vi "Initialize_system.vi"(10 "Serial Port":refnum<visa-resource-name>="COM8", 11 "String in":refnum<vi>) -> (0 "error out":errorcluster, 2 "error?":bool, 3 "VISA Refnum out":refnum<visa-resource-name>, 4 "Results_dir":path)   [LabVIEW 2019]
uses:
  <vilib>/Utility/error.llb/DialogType.ctl
  <vilib>/Instr/_visa.llb/VISA Configure Serial Port (Instr).vi
  Board_Global_Var.vi
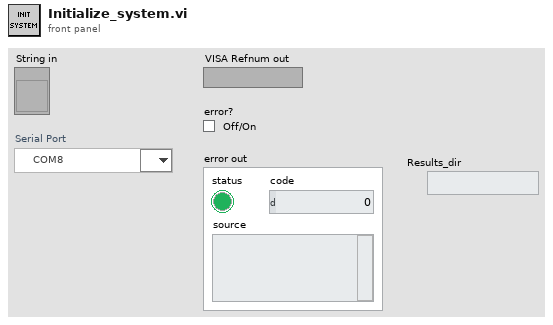
[diagram p1: front panel]
types:
  T1 = typedef "DialogType.ctl" = u16
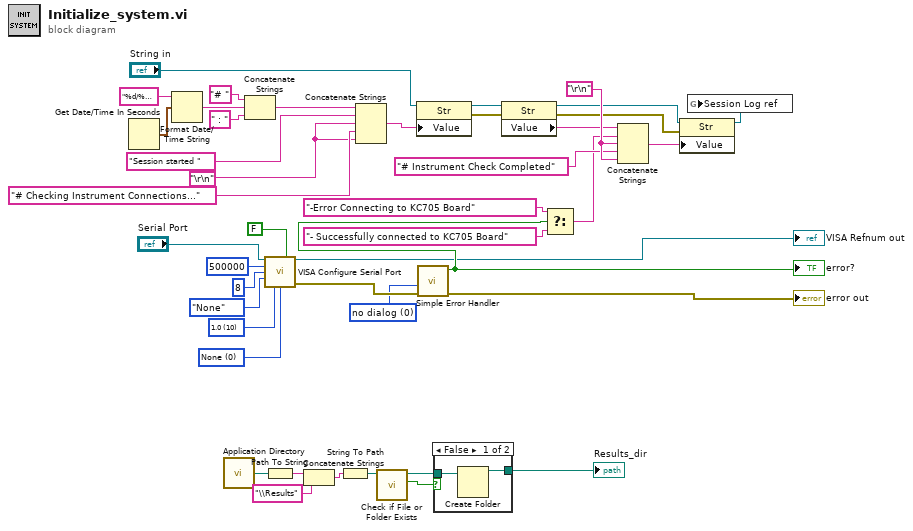
[diagram p0: block diagram]
diagram:
  w34 = u16 0 items=["None", "XON/XOFF", "RTS/CTS", "XON/XOFF & RTS/CTS", "DTR/DSR", "XON/XOFF & DTR/DSR"] ("flow control (0:none)")
  w33 = u16 10 items=["1.0"=10, "1.5"=15, "2.0"=20] ("stop bits (10: 1 bit)")
  w37 = "\r\n"
  w23 = T1 0 items=["no dialog", "OK message", "continue or stop message", "OK message + warnings", "continue/stop + warnings"] ("type of dialog (OK msg:1)")
  w13 = "\r\n"
  n1 = Get Date/Time In Seconds() -> (seconds since 1Jan1904=w19:timestamp)
  n2 = Format Date/Time String(time format string (%c)="%d/%m/%y_%H:%M:%S", seconds (now)=w19) -> (date/time string=w17:string)  [unwired: 1 in]
  n3 = call <vilib>:"Application Directory.vi"() -> ("Application Directory"=w3:path)
  n4 = Concatenate Strings("# " ("string"), w17, " : " ("string")) -> (w16:string)
  n5 = call-poly "VISA Configure Serial Port"("VISA resource name"="Serial Port", "Enable Termination\nChar (T)"=FALSE ("Enable Termination\nChar (T)"), "baud rate (9600)"=u32 500000, "data bits (8)"=u16 8, "parity (0:none)"=enum16{"None", "Odd", "Even", "Mark", "Space"}."None", "stop bits (10: 1 bit)"=w33, "flow control (0:none)"=w34) -> ("VISA resource name out"=→"VISA Refnum out":refnum<visa-resource-name>, "error out"=w38:errorcluster)  [unwired: 7 in]
  n6 = Path To String(path=w3) -> (string=w2:string)
  n7 = Concatenate Strings(w2, "\\Results" ("string")) -> (w8:string)
  n8 = String To Path(string=w8) -> (path=w7:path)
  n9 = Concatenate Strings(w16, "Session started ", w13, "# Checking Instrument Connections..." ("string"), w13) -> (w12:string)
  n10 = call <vilib>:"Check if File or Folder Exists.vi"("path"=w7) -> ("file or folder exists?"=w6:bool, "dup path"=w5:path)  [unwired: 8 in, 1 out]
  n11 = property on="Property Node" class="Str"(reference="String in", "Value"=w12) -> (reference out=w11:refnum<vi>, error out=w10:errorcluster)  [unwired: 1 in]
  n12 = call <vilib>:"Simple Error Handler.vi"("type of dialog (OK msg:1)"=w23, "error in (no error)"=w38) -> ("error?"=w43:bool, "error out"=→"error out":errorcluster)  [unwired: 3 in, 3 out]
  "error?" <- w43
  n13 = case shown="False" w6 {
    tunnel: [w45 w46] -> w1
    tunnel: w5 -> [w44 w46]
    frame False {
      n14 = Create Folder(path (use dialog)=w44) -> (created path=w45:path)  [unwired: 2 in, 2 out]
    }
    frame True {
    }
  }
  "Results_dir" <- w1
  n15 = property on="Property Node" class="Str"(reference=w11, error in=w10) -> (reference out=w28:refnum<vi>, error out=w29:errorcluster, "Value"=w24:string)
  n16 = Select(t="-Error Connecting to KC705 Board" ("string"), s=w43, f="- Successfully connected to KC705 Board" ("string")) -> (s? t:f=w27:string)
  n17 = Concatenate Strings(w24, w27, w37, "# Instrument Check Completed" ("string"), w37) -> (w30:string)
  n18 = property on="Property Node" class="Str"(reference=w28, error in=w29, "Value"=w30) -> (reference out=w31:refnum<vi>)  [unwired: 1 out]
  n19 = global write "Board_Global_Var.vi" "Session Log ref"(w31) -> ()
